vi "change alias and editor properties.vi"(8 "error in":errorcluster, 11 "PL_System Configuration in":refnum<class "NISE_CEF_serializable configuration.lvclass">) -> (0 "error out":errorcluster, 3 "PL_System Configuration out":refnum<class "NISE_CEF_serializable configuration.lvclass">)   [LabVIEW 2013]
uses:
  <vilib>/NI/Configuration Framework/serializable configuration/NISE_CEF_serializable configuration.lvclass
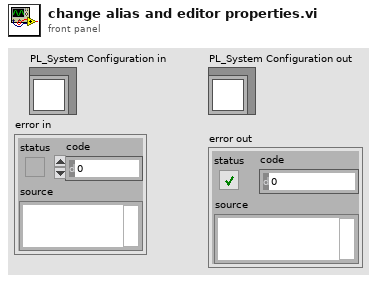
[diagram p1: front panel]
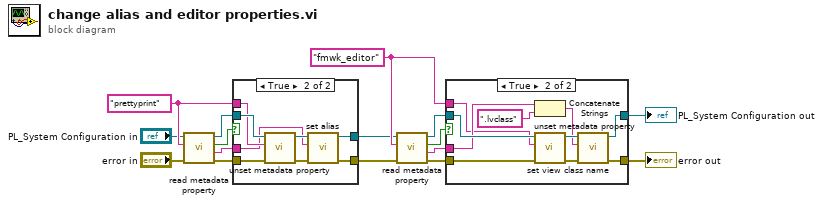
[diagram p0: block diagram]
diagram:
  w15 = "prettyprint" ("key")
  w14 = "fmwk_editor" ("key")
  n1 = call <vilib>:"read metadata property.vi"("error in"="error in", "key"=w15, "configuration in"="PL_System Configuration in") -> ("error out"=w4:errorcluster, "value"=w16:string, "found"=w9:bool, "configuration out"=w3:refnum<class "NISE_CEF_serializable configuration.lvclass">)  [unwired: 5 in]
  n2 = case shown="True" w9 {
    tunnel: w3 -> [w18 w26]
    tunnel: w4 -> [w17 w25]
    tunnel: [w18 w22] -> w5
    tunnel: [w17 w21] -> w6
    tunnel: w15 -> [_ w20]
    tunnel: w16 -> [_ w19]
    frame False {
    }
    frame True {
      n3 = call <vilib>:"unset metadata property.vi"("error in"=w25, "key"=w20, "configuration in"=w26) -> ("error out"=w23:errorcluster, "configuration out"=w24:refnum<class "NISE_CEF_serializable configuration.lvclass">)  [unwired: 7 in]
      n4 = call <vilib>:"set alias.vi"("error in"=w23, "alias"=w19, "configuration in"=w24) -> ("error out"=w21:errorcluster, "configuration out"=w22:refnum<class "NISE_CEF_serializable configuration.lvclass">)  [unwired: 7 in]
    }
  }
  n5 = call <vilib>:"read metadata property.vi"("error in"=w6, "key"=w14, "configuration in"=w5) -> ("error out"=w8:errorcluster, "value"=w13:string, "found"=w11:bool, "configuration out"=w7:refnum<class "NISE_CEF_serializable configuration.lvclass">)  [unwired: 5 in]
  n6 = case shown="True" w11 {
    tunnel: w7 -> [w28 w38]
    tunnel: w8 -> [w27 w37]
    tunnel: [w27 w34] -> w10
    tunnel: [w28 w33] -> w12
    tunnel: w13 -> [_ w32]
    tunnel: w14 -> [_ w29]
    frame False {
    }
    frame True {
      n7 = Concatenate Strings(w32, ".lvclass" ("string")) -> (w30:string)
      n8 = call <vilib>:"unset metadata property.vi"("error in"=w37, "key"=w29, "configuration in"=w38) -> ("error out"=w35:errorcluster, "configuration out"=w36:refnum<class "NISE_CEF_serializable configuration.lvclass">)  [unwired: 7 in]
      n9 = call <vilib>:"set view class name.vi"("error in"=w35, "view class"=w30, "configuration in"=w36) -> ("error out"=w34:errorcluster, "configuration out"=w33:refnum<class "NISE_CEF_serializable configuration.lvclass">)  [unwired: 7 in]
    }
  }
  "PL_System Configuration out" <- w12
  "error out" <- w10
